vi "Create Label Object.vi"(6 "Label Cluster In":T3, 8 "error in (no error)":errorcluster, 9 "Actual Range In":T2, 10 "3D Plot.lvclass in":refnum<class "3D Plot.lvclass">, 11 "Axis Object In":refnum<vi>) -> (0 "error out":errorcluster, 1 "Label Width":T1, 2 "3D Plot.lvclass out":refnum<class "3D Plot.lvclass">, 3 "Axis Object Out":refnum<vi>)   [LabVIEW 2020, in "3D Plot.lvclass"]
uses:
  3D Plot.lvclass
  Tick Array Cluster.ctl
  Tick Array.ctl
  Range Clusters.ctl
  Label Width.ctl
  3D Plot.lvclass/3D Plot.ctl
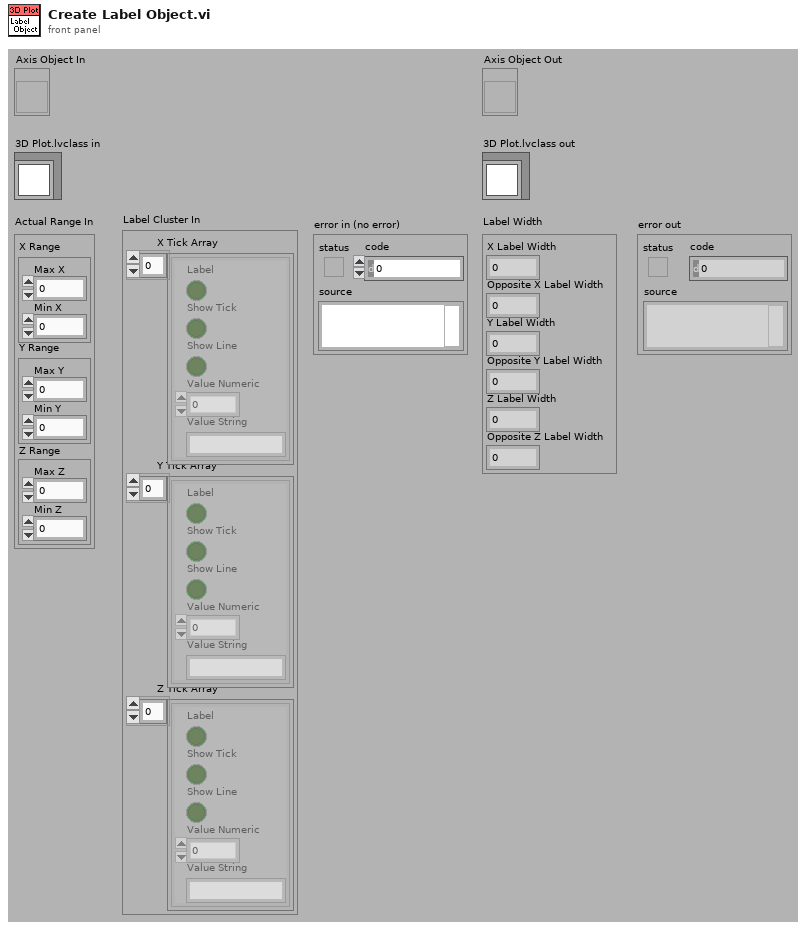
[diagram p1: front panel]
types:
  T1 = typedef "3D Plot.lvclass/Label Width.ctl" = cluster{"X Label Width":sgl, "Opposite X Label Width":sgl, "Y Label Width":sgl, "Opposite Y Label Width":sgl, "Z Label Width":sgl, "Opposite Z Label Width":sgl}
  T2 = typedef "3D Plot.lvclass/Range Clusters.ctl" = cluster{"X Range":cluster{"Max X":sgl, "Min X":sgl}, "Y Range":cluster{"Max Y":sgl, "Min Y":sgl}, "Z Range":cluster{"Max Z":sgl, "Min Z":sgl}}
  T3 = typedef "3D Plot.lvclass/Tick Array Cluster.ctl" = cluster{"X Tick Array":T4, "Y Tick Array":T4, "Z Tick Array":T4}
  T4 = typedef "3D Plot.lvclass/Tick Array.ctl" = cluster{"Label":bool, "Show Tick":bool, "Show Line":bool, "Value Numeric":sgl, "Value String":string}[]
  T5 = enum16{"X", "Y", "Z", "X Opposite", "Y Opposite", "Z Opposite"}
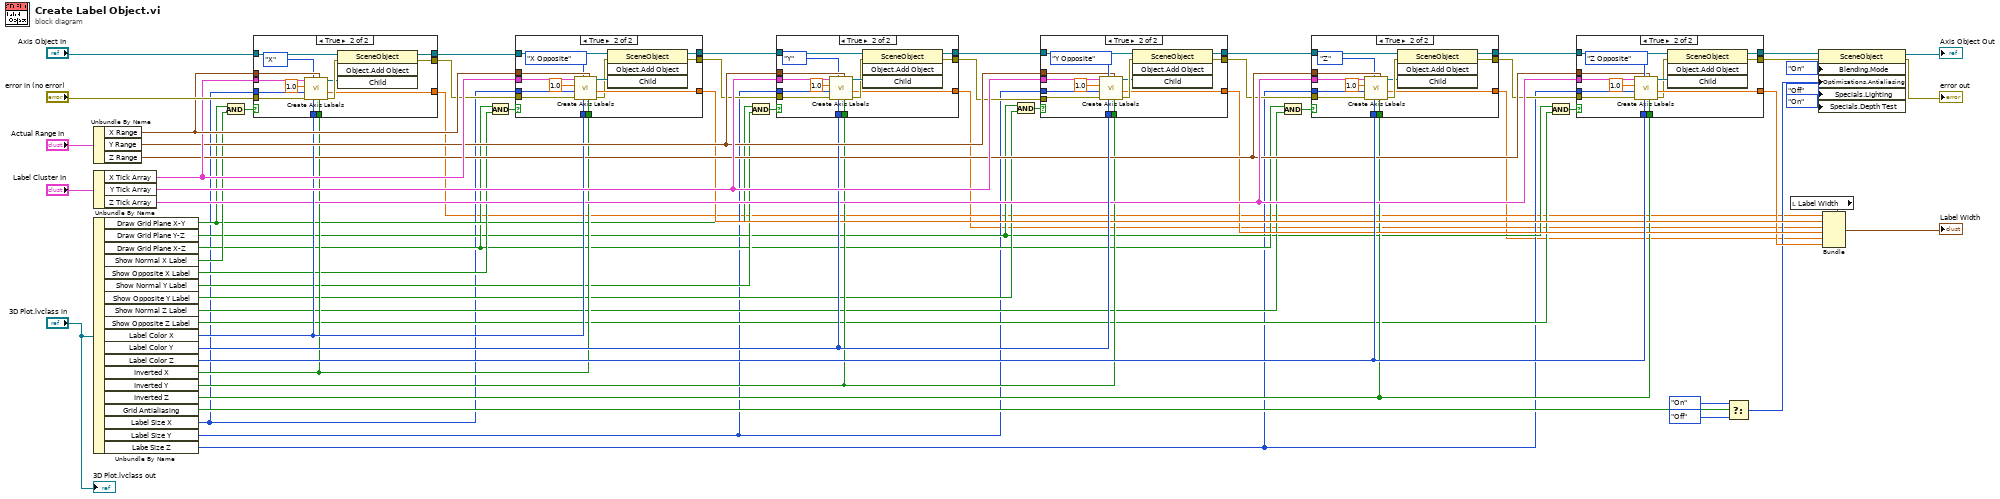
[diagram p0: block diagram]
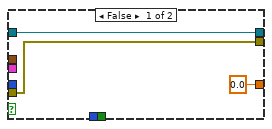
[diagram p2: hidden frame]
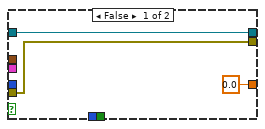
[diagram p3: hidden frame]
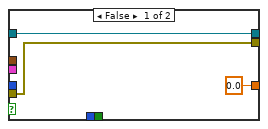
[diagram p4: hidden frame]
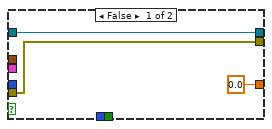
[diagram p5: hidden frame]
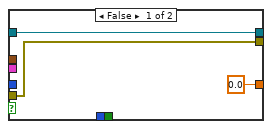
[diagram p6: hidden frame]
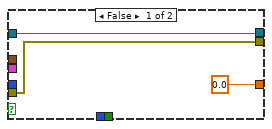
[diagram p7: hidden frame]
diagram:
  n1 = Unbundle By Name("Actual Range In") -> ("X Range"=w56:cluster{"Max X":sgl, "Min X":sgl}, "Y Range"=w53:cluster{"Max Y":sgl, "Min Y":sgl}, "Z Range"=w48:cluster{"Max Z":sgl, "Min Z":sgl})
  n2 = Unbundle By Name("Label Cluster In") -> ("X Tick Array"=w55:T4, "Y Tick Array"=w54:T4, "Z Tick Array"=w49:T4)
  n3 = Unbundle By Name("3D Plot.lvclass in") -> ("Draw Grid Plane X-Y"=w28:bool, "Draw Grid Plane Y-Z"=w21:bool, "Draw Grid Plane X-Z"=w24:bool, "Show Normal X Label"=w31:bool, "Show Opposite X Label"=w30:bool, "Show Normal Y Label"=w27:bool, "Show Opposite Y Label"=w26:bool, "Show Normal Z Label"=w23:bool, "Show Opposite Z Label"=w22:bool, "Label Color X"=w52:u32, "Label Color Y"=w51:u32, "Label Color Z"=w50:u32, "Inverted X"=w37:bool, "Inverted Y"=w39:bool, "Inverted Z"=w38:bool, "Grid Antialiasing"=w12:bool, "Label Size X"=w9:u16, "Label Size Y"=w8:u16, "Labe Size Z"=w7:u16)
  n4 = And(x=w28, y=w31) -> (x .and. y?=w5:bool)
  n5 = case shown="True" w5 {
    tunnel: "Axis Object In" -> [w67 w81]
    tunnel: "error in (no error)" -> [w66 w80]
    tunnel: w56 -> [_ w79]
    tunnel: w55 -> [_ w78]
    tunnel: w52 -> [_ w77]
    tunnel: [w67 w76] -> w47
    tunnel: w37 -> [_ w75]
    tunnel: [w66 w74] -> w36
    tunnel: w9 -> [_ w73]
    tunnel: [sgl 0.0 w68] -> w6
    frame False {
    }
    frame True {
      n6 = call "Create Axis Labels.vi"("Inverted"=w75, "Range"=w79, "Font Color"=w77, "Which Axis?"=T5."X", "error in (no error)"=w80, "Font Size"=w73, "Alpha"=sgl 1.0, "Tick Cluster Array"=w78) -> ("error out"=w71:errorcluster, "Max Width"=w68:sgl, "New Label Object"=w70:refnum<vi>)  [unwired: 1 out]
      n7 = invoke class="SceneObject" method="Object.Add Object"(reference=w81, error in=w71, "Child"=w70) -> (reference out=w76:refnum<vi>, error out=w74:errorcluster)  [unwired: 1 in, 2 out]
    }
  }
  n8 = And(x=w24, y=w30) -> (x .and. y?=w29:bool)
  n9 = case shown="True" w29 {
    tunnel: w55 -> [_ w93]
    tunnel: w56 -> [_ w95]
    tunnel: w52 -> [_ w87]
    tunnel: w47 -> [w84 w98]
    tunnel: [sgl 0.0 ("Max Width") w89] -> w42
    tunnel: [w84 w97] -> w46
    tunnel: w9 -> [_ w92]
    tunnel: w37 -> [_ w86]
    tunnel: w36 -> [w82 w91]
    tunnel: [w82 w96] -> w35
    frame False {
    }
    frame True {
      n10 = call "Create Axis Labels.vi"("Inverted"=w86, "Range"=w95, "Font Color"=w87, "Which Axis?"=T5."X Opposite", "error in (no error)"=w91, "Font Size"=w92, "Alpha"=sgl 1.0, "Tick Cluster Array"=w93) -> ("error out"=w88:errorcluster, "Max Width"=w89:sgl, "New Label Object"=w90:refnum<vi>)  [unwired: 1 out]
      n11 = invoke class="SceneObject" method="Object.Add Object"(reference=w98, error in=w88, "Child"=w90) -> (reference out=w97:refnum<vi>, error out=w96:errorcluster)  [unwired: 1 in, 2 out]
    }
  }
  n12 = And(x=w28, y=w27) -> (x .and. y?=w3:bool)
  n13 = case shown="True" w3 {
    tunnel: w54 -> [_ w115]
    tunnel: w53 -> [_ w114]
    tunnel: w51 -> [_ w113]
    tunnel: w46 -> [w101 w112]
    tunnel: [w101 w111] -> w45
    tunnel: w39 -> [_ w110]
    tunnel: w35 -> [w100 w109]
    tunnel: [w100 w108] -> w34
    tunnel: w8 -> [_ w107]
    tunnel: [sgl 0.0 ("Max Width") w103] -> w4
    frame False {
    }
    frame True {
      n14 = call "Create Axis Labels.vi"("Inverted"=w110, "Range"=w114, "Font Color"=w113, "Which Axis?"=T5."Y", "error in (no error)"=w109, "Font Size"=w107, "Alpha"=sgl 1.0, "Tick Cluster Array"=w115) -> ("error out"=w104:errorcluster, "Max Width"=w103:sgl, "New Label Object"=w105:refnum<vi>)  [unwired: 1 out]
      n15 = invoke class="SceneObject" method="Object.Add Object"(reference=w112, error in=w104, "Child"=w105) -> (reference out=w111:refnum<vi>, error out=w108:errorcluster)  [unwired: 1 in, 2 out]
    }
  }
  n16 = And(x=w21, y=w26) -> (x .and. y?=w25:bool)
  n17 = case shown="True" w25 {
    tunnel: w54 -> [_ w127]
    tunnel: w53 -> [_ w128]
    tunnel: w51 -> [_ w124]
    tunnel: w45 -> [w118 w132]
    tunnel: [sgl 0.0 ("Max Width") w121] -> w41
    tunnel: [w118 w131] -> w44
    tunnel: w8 -> [_ w126]
    tunnel: w39 -> [_ w123]
    tunnel: w34 -> [w116 w125]
    tunnel: [w116 w130] -> w33
    frame False {
    }
    frame True {
      n18 = call "Create Axis Labels.vi"("Inverted"=w123, "Range"=w128, "Font Color"=w124, "Which Axis?"=T5."Y Opposite", "error in (no error)"=w125, "Font Size"=w126, "Alpha"=sgl 1.0, "Tick Cluster Array"=w127) -> ("error out"=w122:errorcluster, "Max Width"=w121:sgl, "New Label Object"=w120:refnum<vi>)  [unwired: 1 out]
      n19 = invoke class="SceneObject" method="Object.Add Object"(reference=w132, error in=w122, "Child"=w120) -> (reference out=w131:refnum<vi>, error out=w130:errorcluster)  [unwired: 1 in, 2 out]
    }
  }
  n20 = And(x=w24, y=w23) -> (x .and. y?=w1:bool)
  n21 = case shown="True" w1 {
    tunnel: w50 -> [_ w149]
    tunnel: w49 -> [_ w148]
    tunnel: w48 -> [_ w147]
    tunnel: w44 -> [w135 w146]
    tunnel: [w135 w145] -> w43
    tunnel: w38 -> [_ w144]
    tunnel: w33 -> [w134 w143]
    tunnel: [w134 w142] -> w32
    tunnel: w7 -> [_ w141]
    tunnel: [sgl 0.0 ("Max Width") w137] -> w2
    frame False {
    }
    frame True {
      n22 = call "Create Axis Labels.vi"("Inverted"=w144, "Range"=w147, "Font Color"=w149, "Which Axis?"=T5."Z", "error in (no error)"=w143, "Font Size"=w141, "Alpha"=sgl 1.0, "Tick Cluster Array"=w148) -> ("error out"=w140:errorcluster, "Max Width"=w137:sgl, "New Label Object"=w139:refnum<vi>)  [unwired: 1 out]
      n23 = invoke class="SceneObject" method="Object.Add Object"(reference=w146, error in=w140, "Child"=w139) -> (reference out=w145:refnum<vi>, error out=w142:errorcluster)  [unwired: 1 in, 2 out]
    }
  }
  n24 = And(x=w21, y=w22) -> (x .and. y?=w20:bool)
  n25 = case shown="True" w20 {
    tunnel: w49 -> [_ w156]
    tunnel: w48 -> [_ w162]
    tunnel: w50 -> [_ w155]
    tunnel: w43 -> [w152 w166]
    tunnel: [sgl 0.0 ("Max Width") w160] -> w40
    tunnel: [w152 w165] -> w16
    tunnel: w7 -> [_ w157]
    tunnel: w38 -> [_ w154]
    tunnel: w32 -> [w150 w158]
    tunnel: [w150 w164] -> w11
    frame False {
    }
    frame True {
      n26 = call "Create Axis Labels.vi"("Inverted"=w154, "Range"=w162, "Font Color"=w155, "Which Axis?"=T5."Z Opposite", "error in (no error)"=w158, "Font Size"=w157, "Alpha"=sgl 1.0, "Tick Cluster Array"=w156) -> ("error out"=w159:errorcluster, "Max Width"=w160:sgl, "New Label Object"=w161:refnum<vi>)  [unwired: 1 out]
      n27 = invoke class="SceneObject" method="Object.Add Object"(reference=w166, error in=w159, "Child"=w161) -> (reference out=w165:refnum<vi>, error out=w164:errorcluster)  [unwired: 1 in, 2 out]
    }
  }
  n28 = Select(t=enum16{"Inherit Value", "Off", "On"}."On" ("Optimizations:Antialiasing"), s=w12, f=enum16{"Inherit Value", "Off", "On"}."Off" ("Optimizations:Antialiasing")) -> (s? t:f=w13:enum16{"Inherit Value", "Off", "On"})
  n29 = local read "Label Width"() -> (w10:T1)
  n30 = property class="SceneObject"(reference=w16, error in=w11, "Blending.Mode"=enum16{"Inherit Value", "Off", "On"}."On" ("Specials:Lighting"), "Optimizations.Antialiasing"=w13, "Specials.Lighting"=enum16{"Inherit Value", "Off", "On"}."Off" ("Blending:Mode"), "Specials.Depth Test"=enum16{"Inherit Value", "Off", "On"}."On" ("Specials:Depth Test")) -> (reference out=→"Axis Object Out":refnum<vi>, error out=→"error out":errorcluster)
  n31 = Bundle(cluster=w10, "X Label Width"=w6, "Opposite X Label Width"=w42, "Y Label Width"=w4, "Opposite Y Label Width"=w41, "Z Label Width"=w2, "Opposite Z Label Width"=w40) -> (→"Label Width":T1)
  "3D Plot.lvclass out" <- "3D Plot.lvclass in"
